vi "Serialize.vi"(8 "error in (no error)":errorcluster, 11 "VIPB Build in":refnum<class "VIPB Build.lvclass">) -> (0 "error out":errorcluster, 2 "Text":string)   [LabVIEW 2014, in "VIPB Build.lvclass"]
uses:
  VIPB Build.lvclass
  Shared/Controls/VIPB Build - STYP.ctl
  VIPB Build.lvclass/VIPB Build.ctl
  Read Install after build.vi
  Read LV Version.vi
  Read VIPB_Path.vi
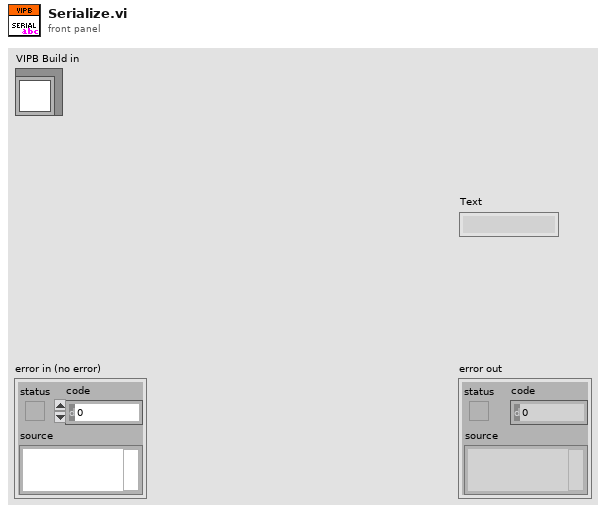
[diagram p1: front panel]
types:
  T1 = typedef "VIPB Build - STYP.ctl" = cluster{"VIPB Path":string, "Install after build":bool, "LabVIEW Version":string}
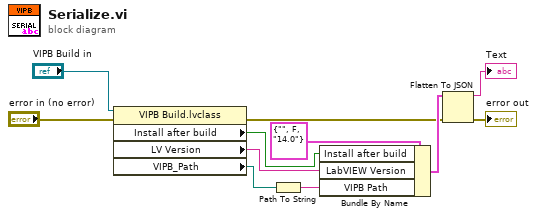
[diagram p0: block diagram]
diagram:
  n1 = property class="VIPB Build.lvclass"(reference="VIPB Build in", error in="error in (no error)") -> (error out=w3:errorcluster, "Install after build"=w8:bool, "LV Version"=w7:string, "VIPB_Path"=w6:path)  [unwired: 1 out]
  n2 = Path To String(path=w6) -> (string=w5:string)
  n3 = Bundle By Name(cluster=T1 {"VIPB Path"="", "Install after build"=FALSE, "LabVIEW Version"="14.0"} ("VIPB Build"), "Install after build"=w8, "LabVIEW Version"=w7, "VIPB Path"=w5) -> (w4:T1)
  n4 = Flatten To JSON(anything=w4, error in (no error)=w3) -> (JSON string=→"Text":string, 11:→"error out":errorcluster)  [unwired: 1 in]
